vi "Network Engine.vi"(8 "error in (no error)":errorcluster, 11 "Variables":T1={"Process Ref"=refnum, "Comm Ref"=refnum, "Data Refs"={"ProtectionsAndCounters.Ref"=refnum, "Signals.Ref"=refnum, "Status.Ref"=refnum, "Overrides"=refnum, "IncomingSignals.Ref"=refnum, "CtrandProtctnVld.Ref"=refnum, "RcvTime.Ref"=refnum, "TimeDiff.Ref"=refnum, "IncomingProtCtr.Ref"=refnum}, "Settings"={"Name"="", "Priority"=0, "XNET Settings"={"Database"="", "Cluster"="", "Port"="", "Baud rate [Bd]"=0, "Termination"=0, "CAN I/O Mode"=0, "FD Baud rate [Bd]"=500000, "Priority"=100, "Use Legacy"=FALSE, "FD ISO Mode"=0}, "FPGA Session"=0, "Outgoing CAN Session"="", "Outgoing Frame Count"=0, "Outgoing Frames"=[], "Incoming CAN Session"="", "Incoming Frame Count"=0, "Incoming Frames"=[], "Incoming Frame IDs"=[], "Incoming Frame Timestamp"=[], "Incoming Values"={"Signal Values"=[], "Signal_Invalid_Values"=[], "ProtCtr Sig Values"=[]}}, "Stream Refs"={"Addon"="", "Port"="", "Filter Ref"=refnum, "Default Filter"={"ID Filters"=[], "Direction Filter"=enum."Tx/Rx", "Type Filter"=enum."All"}, "Port Settings"={"Mode"=0, "Baud Rate"=0, "Termination"=0, "FD ISO Mode"=0, "FD Baud Rate"=0}}} {"Stream Refs"."Port Settings"."FD ISO Mode" items=["ISO", "Non ISO", "ISO Legacy"]; "Stream Refs"."Port Settings"."Termination" items=["Off", "On"]; "Stream Refs"."Port Settings"."Mode" items=["CAN 2.0", "CAN FD", "CAN FD+BRS"]; "Settings"."XNET Settings"."FD ISO Mode" items=["ISO", "Non ISO", "ISO Legacy"]; "Settings"."XNET Settings"."CAN I/O Mode" items=["CAN 2.0", "CAN FD", "CAN FD+BRS"]; "Settings"."XNET Settings"."Termination" items=["Off", "On"]}) -> (0 "error out":errorcluster)   [LabVIEW 2019, in "Protection and Counter Addon Engine.lvlib"]
uses:
  Protection and Counter Addon Engine.lvlib
  Types/RT Async Engine Variables.ctl
  <vilib>/NI/NIVS Inline Async API/_VS Inline Async API/Process/Process.lvclass
  <vilib>/NI/NI VeriStand Addon Network Comm/Engine/VeriStand Comm.lvclass
  Types/RT Data References.ctl
  <vilib>/NI/NIVS Inline Async API/_Data Access Engine/Data Access Engine/Types/Write.DVR.ctl
  <vilib>/NI/NIVS Inline Async API/_Data Access Engine/Access Type Classes/Write/Write.lvclass
  <vilib>/NI/NIVS Inline Async API/_Data Access Engine/Data Access Engine/Types/Read.DVR.ctl
  <vilib>/NI/NIVS Inline Async API/_Data Access Engine/Access Type Classes/Read/Read.lvclass
  Types/RT Async Engine Settings.ctl
  Addon Shared/Types/XNET Settings.ctl
  SubModules/Frame-Protection-Support/Source/Engine/Types/RT Frame Settings.ctl
  SubModules/Frame-Protection-Support/Source/Shared/Types/Exported Frame Type.ctl
  SubModules/Frame-Protection-Support/Source/Engine/Types/RT Protection Configuration.ctl
  SubModules/Frame-Protection-Support/Source/Shared/Types/Protection Type.ctl
  SubModules/Frame-Protection-Support/Source/Shared/Types/XNET Signal Configuration.ctl
  SubModules/Frame-Protection-Support/Source/Shared/Types/Exported Counter Settings.ctl
  SubModules/Frame-Protection-Support/Source/Shared/Types/Exported Event Trigger Type.ctl
  Types/Incoming Values.ctl
  SubModules/CAN-Streaming-Support/Source/Addon/Addon Engine/Types/Engine Stream Refs.ctl
  SubModules/CAN-Streaming-Support/Source/Addon/Addon Shared/Types/Direction Filter.ctl
  SubModules/CAN-Streaming-Support/Source/Addon/Addon Shared/Types/Type Filter.ctl
  SubModules/CAN-Streaming-Support/Source/Addon/Addon Shared/Types/Filter Parameters.ctl
  SubModules/CAN-Streaming-Support/Source/Addon/Addon Engine/Types/Engine Stream Port Settings.ctl
  <vilib>/NI/NI VeriStand Addon Network Comm/Engine/VeriStand Comm.lvclass/VeriStand Comm.ctl
  <vilib>/NI/NIVS Inline Async API/_VS Inline Async API/Process/Process.lvclass/Process.ctl
  <vilib>/xnet/xnet.llb/XNET Frame CAN.ctl
  <vilib>/xnet/xnet.llb/XNET Frame Type CAN.ctl
  <vilib>/NI/NI VeriStand Addon Network Comm/Engine/_SubVIs/Comm Connection Engine.vi
  <vilib>/NI/NI VeriStand Addon Network Comm/Engine/_SubVIs/Comm Command Engine.vi
  <vilib>/NI/NIVS Inline Async API/_VS Inline Async API/Error Handling Process/SubVIs/Error.ConvertArray.vi
  <vilib>/NI/AMC/Read Next Message.vi
  <vilib>/NI/Tools/Keyed Array/Index.vi
  <vilib>/NI/AMC/Send Local Message.vi
  <vilib>/NI/STM/Connection Manager/TCP/Advanced/TCP Connection Manager (By Reference).vi
  <vilib>/Utility/error.llb/Clear Errors.vi
  <vilib>/NI/STM/Get Connection Reference.vi
  <vilib>/NI/STM/TCP/Get Connection Reference (TCP).vi
  <vilib>/NI/STM/Read Meta Data.vi
  <vilib>/NI/STM/TCP/Read Meta Data (TCP Ref).vi
  <vilib>/NI/Tools/Keyed Array/Add.vi
  <vilib>/NI/STM/Connection Manager/TCP/Advanced/TCP Check Connection (By Reference).vi
  <vilib>/NI/AMC/Read Termination Message.vi
  <vilib>/NI/Tools/Keyed Array/Map String.vi
  <vilib>/NI/AMC/Create Single Message.vi
  <vilib>/NI/AMC/Update Message Routing Info.vi
  <vilib>/NI/STM/SubVIs/Generate STM Error.vi
  <vilib>/NI/Tools/String/Get Case Matching.vi
  <vilib>/NI/STM/Read Message.vi
  <vilib>/NI/STM/TCP/Read Message (TCP).vi
  <vilib>/NI/AMC/Send Message.vi
  <vilib>/NI/NI VeriStand Addon Network Comm/Shared/Comm Constants.vi
  <vilib>/NI/AMC/Create Message Queue.vi
  <vilib>/NI/AMC/Globals.vi
  <vilib>/NI/STM/Write Message.vi
  <vilib>/NI/STM/TCP/Write Message (TCP).vi
  <vilib>/NI/AMC/Destroy Message Queue.vi
  <vilib>/Utility/SystemLogging/Write to System Log.vi
  <vilib>/NI/STM/TCP/Read Meta Data (TCP Clst).vi
  <vilib>/xnet/xnet.llb/XNET Write (Frame CAN).vi
  SubModules/CAN-Streaming-Support/Source/Addon/Addon Engine/CAN Stream Support Engine.lvlib
  SubModules/CAN-Streaming-Support/Source/Addon/Addon Shared/CAN Stream Support Shared.lvlib
  SubModules/Frame-Protection-Support/Source/Shared/Protection and Counter Support Shared.lvlib
  SubModules/Frame-Protection-Support/Source/Engine/Protection and Counter Support Engine.lvlib
  <vilib>/NI/NIVS Inline Async API/_Data Access Engine/Data Access Engine/Data Access Engine.lvclass
  Addon Shared/Protection and Counter Addon Shared.lvlib
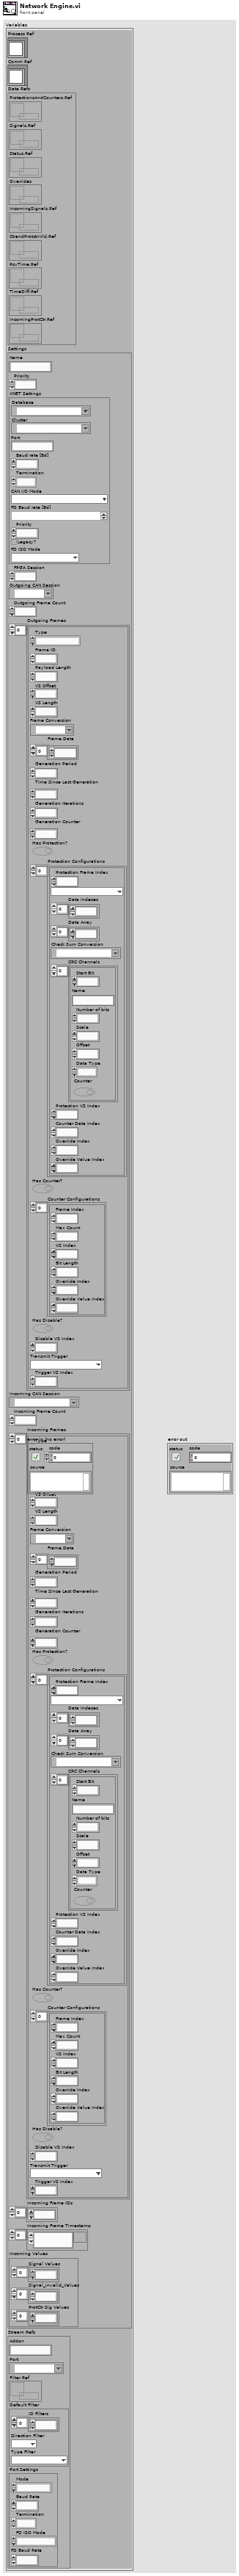
[diagram p1: front panel]
types:
  T1 = typedef "Protection and Counter Addon Engine.lvlib/RT Async Engine Variables.ctl" = cluster{"Process Ref":refnum<class "Process.lvclass">, "Comm Ref":refnum<class "VeriStand Comm.lvclass">, "Data Refs":T2, "Settings":T5, "Stream Refs":T15}
  T2 = typedef "Protection and Counter Addon Engine.lvlib/RT Data References.ctl" = cluster{"ProtectionsAndCounters.Ref":T3, "Signals.Ref":T4, "Status.Ref":T3, "Overrides":T4, "IncomingSignals.Ref":T3, "CtrandProtctnVld.Ref":T3, "RcvTime.Ref":T3, "TimeDiff.Ref":T3, "IncomingProtCtr.Ref":T3}
  T3 = typedef "Data Access Engine.lvlib/Data Access Engine.lvclass/Write.DVR.ctl" = refnum<data-value>
  T4 = typedef "Data Access Engine.lvlib/Data Access Engine.lvclass/Read.DVR.ctl" = refnum<data-value>
  T5 = typedef "Protection and Counter Addon Engine.lvlib/RT Async Engine Settings.ctl" = cluster{"Name":string, "Priority":i32, "XNET Settings":T6, "FPGA Session":u32, "Outgoing CAN Session":refnum<k21>, "Outgoing Frame Count":i32, "Outgoing Frames":T7[], "Incoming CAN Session":refnum<k21>, "Incoming Frame Count":i32, "Incoming Frames":T7[], "Incoming Frame IDs":u32[], "Incoming Frame Timestamp":timestamp[], "Incoming Values":T14}
  T6 = typedef "Protection and Counter Addon Shared.lvlib/XNET Settings.ctl" = cluster{"Database":refnum<k21>, "Cluster":refnum<k21>, "Port":string, "Baud rate [Bd]":u64, "Termination":u32, "CAN I/O Mode":u32, "FD Baud rate [Bd]":u64, "Priority":i32, "Use Legacy":bool, "FD ISO Mode":u32}
  T7 = typedef "Protection and Counter Support Engine.lvlib/RT Frame Settings.ctl" = cluster{"Type":T8, "Frame ID":u32, "Payload Length":u32, "VS Offset":i32, "VS Length":i32, "Frame Conversion":refnum<k21>, "Frame.Data":dbl[], "Generation Period":u32, "Time Since Last Generation":u32, "Generation Iterations":u32, "Generation Counter":u32, "Has Protection?":bool, "Protection Configurations":T9[], "Has Counter?":bool, "Counter Configurations":T12[], "Has Disable?":bool, "Disable VS Index":i32, "Transmit Trigger":T13, "Trigger VS Index":i32}
  T8 = typedef "Protection and Counter Support Shared.lvlib/Exported Frame Type.ctl" = enum16{"Periodic", "Event", "Periodic/Event"}
  T9 = typedef "Protection and Counter Support Engine.lvlib/RT Protection Configuration.ctl" = cluster{"Protection Frame Index":i32, "Protection Type":T10, "Data Indeces":i32[], "Data Array":dbl[], "Check Sum Conversion":refnum<k21>, "CRC Channels":T11[], "Protection VS Index":i32, "Counter Data Index":i32, "Override Index":i32, "Override Value Index":i32}
  T10 = typedef "Protection and Counter Support Shared.lvlib/Protection Type.ctl" = enum16{"Arb ID + Bytes Checksum with Inversion", "Arb ID + Bytes CRC with Inversion", "Reversed Raw Signal Checksum with Inversion", "Concatenated Two's Compliment"}
  T11 = typedef "Protection and Counter Support Shared.lvlib/XNET Signal Configuration.ctl" = cluster{"Start Bit":i32, "Name":string, "Number of bits":i32, "Scale":dbl, "Offset":dbl, "Data Type":u32, "Counter":bool}
  T12 = typedef "Protection and Counter Support Shared.lvlib/Exported Counter Settings.ctl" = cluster{"Frame Index":i32, "Max Count":dbl, "VS Index":i32, "Bit Length":i64, "Override Index":i32, "Override Value Index":i32}
  T13 = typedef "Protection and Counter Support Shared.lvlib/Exported Event Trigger Type.ctl" = enum16{"Channel value change", "Trigger channel (not zero)", "Channel value change or trigger channel (not zero)", "Trigger channel (any value change)", "Channel value change or trigger channel (any value change)"}
  T14 = typedef "Protection and Counter Addon Engine.lvlib/Incoming Values.ctl" = cluster{"Signal Values":dbl[], "Signal_Invalid_Values":dbl[], "ProtCtr Sig Values":dbl[]}
  T15 = typedef "CAN Stream Support Engine.lvlib/Engine Stream Refs.ctl" = cluster{"Addon":string, "Port":refnum<k21>, "Filter Ref":refnum<data-value>, "Default Filter":T16, "Port Settings":T19}
  T16 = typedef "CAN Stream Support Shared.lvlib/Filter Parameters.ctl" = cluster{"ID Filters":u32[], "Direction Filter":T17, "Type Filter":T18}
  T17 = typedef "CAN Stream Support Shared.lvlib/Direction Filter.ctl" = enum16{"Tx/Rx", "Rx", "Tx"}
  T18 = typedef "CAN Stream Support Shared.lvlib/Type Filter.ctl" = enum16{"All", "CAN Data", "CAN Remote", "CAN Bus Error", "CAN 2.0 Data", "CAN FD Data", "CAN FD+BRS Data", "J1939 Data", "Delay", "Log Trigger", "Start Trigger"}
  T19 = typedef "CAN Stream Support Engine.lvlib/Engine Stream Port Settings.ctl" = cluster{"Mode":u32, "Baud Rate":u64, "Termination":u32, "FD ISO Mode":u32, "FD Baud Rate":u64}
  T20 = typedef "XNET Frame CAN.ctl" = cluster{"timestamp":timestamp, "payload":u8[], "identifier":u32, "type":T21, "extended?":bool, "echo?":bool}
  T21 = typedef "XNET Frame Type CAN.ctl" = u8
  T22 = typedef "NI VeriStand Addon Network Comm.lvlib/VeriStand Comm.lvclass/Response Information.ctl" = cluster{"response name":string, "responseQ":string}
  T23 = cluster{"ID Filters":u32[], "Direction Filter":T17, "Type Filter":T18}
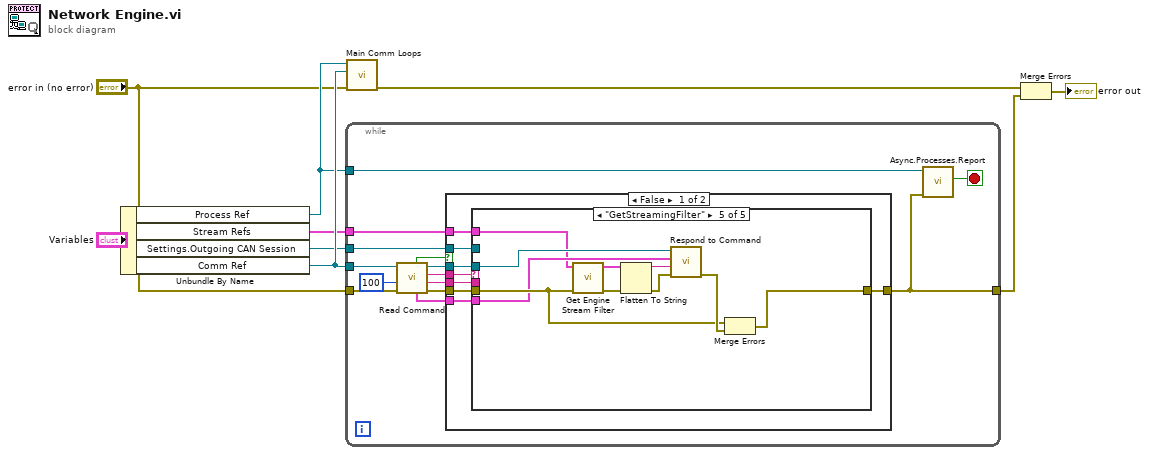
[diagram p0: block diagram]
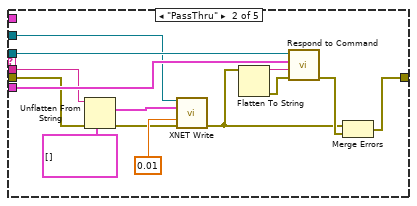
[diagram p3: hidden frame]
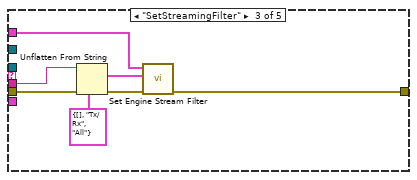
[diagram p4: hidden frame]
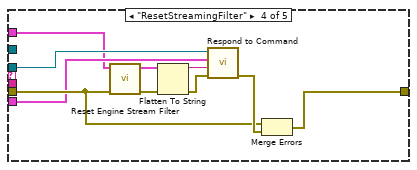
[diagram p5: hidden frame]
diagram:
  n1 = Unbundle By Name("Variables") -> ("Process Ref"=w4:refnum<class "Process.lvclass">, "Stream Refs"=w1:T15, "Settings.Outgoing CAN Session"=w5:refnum<k21>, "Comm Ref"=w6:refnum<class "VeriStand Comm.lvclass">)
  n2 = while {
    tunnel: w4 -> [w23]
    tunnel: "error in (no error)" -> [w21]
    tunnel: w6 -> [w20]
    tunnel: w5 -> [w17]
    tunnel: [w14] -> w7
    tunnel: w1 -> [w10]
    stop <- w22 stop-if-true
    n3 = call <vilib>:"Read Command.vi"("error in (no error)"=w21, "timeout (100 ms)"=100, "VeriStand Comm in"=w20) -> ("error out"=w15:errorcluster, "message value"=w16:string, "message name"=w13:string, "VeriStand Comm out"=w19:refnum<class "VeriStand Comm.lvclass">, "ResponseInfo"=w18:T22, "timed out?"=w12:bool)  [unwired: 3 in]
    n4 = case shown="False" w12 {
      tunnel: w19 -> [w31 _]
      tunnel: w18 -> [w30 _]
      tunnel: w17 -> [w29 _]
      tunnel: w16 -> [w28 _]
      tunnel: w15 -> [w27 w74]
      tunnel: [w26 w74] -> w14
      tunnel: w13 -> [w25 _]
      tunnel: w10 -> [w24 _]
      frame False {
        n5 = case shown="\"GetStreamingFilter\"" w25 {
          tunnel: w31 -> [_ w46 _ w56 w66]
          tunnel: w30 -> [_ w45 _ w55 w65]
          tunnel: w29 -> [_ w43 _ _ _]
          tunnel: w28 -> [_ w42 w53 _ _]
          tunnel: w27 -> [w32 w41 w51 w58 w68]
          tunnel: [w32 w36 w48 w57 w67] -> w26
          tunnel: w24 -> [_ _ w47 w54 w64]
          frame "", Default {
          }
          frame "PassThru" {
            n6 = Unflatten From String(type=T20[] [] ("data"), binary string=w42, error in (no error)=w41) -> (value=w38:T20[], error out=w40:errorcluster)  [unwired: 2 in, 1 out]
            n7 = call-poly <vilib>:"XNET Write.vi"("session in"=w43, "data"=w38, "timeout (10)"=0.01, "error in (no error)"=w40) -> ("error out"=w34:errorcluster)  [unwired: 10 in, 1 out]
            n8 = Flatten To String(anything=w34) -> (data string=w35:string, error out=w33:errorcluster)  [unwired: 3 in, 1 out]
            n9 = call <vilib>:"Respond to Command.vi"("error in (no error)"=w33, "message value"=w35, "ResponseInfo"=w45, "VeriStand Comm in"=w46) -> ("error out"=w37:errorcluster)  [unwired: 5 in, 2 out]
            n10 = Merge Errors(w34, w37) -> (w36:errorcluster)
          }
          frame "SetStreamingFilter" {
            n11 = Unflatten From String(type=T16 {"ID Filters"=[], "Direction Filter"=enum."Tx/Rx", "Type Filter"=enum."All"} ("Filter"), binary string=w53, error in (no error)=w51) -> (value=w49:T16, error out=w52:errorcluster)  [unwired: 2 in, 1 out]
            n12 = call "Set Engine Stream Filter.vi"("error in (no error)"=w52, "Filter"=w49, "Refs"=w47) -> ("error out"=w48:errorcluster)  [unwired: 8 in]
          }
          frame "ResetStreamingFilter" {
            n13 = call "Reset Engine Stream Filter.vi"("error in (no error)"=w58, "Refs"=w54) -> ("error out"=w59:errorcluster, "Filter"=w60:T16)  [unwired: 8 in]
            n14 = Flatten To String(anything=w60, error in (no error)=w59) -> (data string=w62:string, error out=w61:errorcluster)  [unwired: 2 in, 1 out]
            n15 = call <vilib>:"Respond to Command.vi"("error in (no error)"=w61, "message value"=w62, "ResponseInfo"=w55, "VeriStand Comm in"=w56) -> ("error out"=w63:errorcluster)  [unwired: 5 in, 2 out]
            n16 = Merge Errors(w58, w63) -> (w57:errorcluster)
          }
          frame "GetStreamingFilter" {
            n17 = call "Get Engine Stream Filter.vi"("error in (no error)"=w68, "Refs"=w64) -> ("error out"=w69:errorcluster, "Filter"=w70:T23)  [unwired: 8 in]
            n18 = Flatten To String(anything=w70, error in (no error)=w69) -> (data string=w72:string, error out=w71:errorcluster)  [unwired: 2 in, 1 out]
            n19 = call <vilib>:"Respond to Command.vi"("error in (no error)"=w71, "message value"=w72, "ResponseInfo"=w65, "VeriStand Comm in"=w66) -> ("error out"=w73:errorcluster)  [unwired: 5 in, 2 out]
            n20 = Merge Errors(w68, w73) -> (w67:errorcluster)
          }
        }
      }
      frame True {
      }
    }
    n21 = call <vilib>:"Async.Processes.Report.vi"("Error"=w14, "Process in"=w23) -> ("Stop"=w22:bool)  [unwired: 8 in, 1 out]
  }
  n22 = call <vilib>:"Main Comm Loops.vi"("error in (no error)"="error in (no error)", "Comm.lvclass"=w6, "Process"=w4) -> ("error out"=w8:errorcluster)  [unwired: 8 in]
  n23 = Merge Errors(w8, w7) -> (→"error out":errorcluster)
